vi "send load from string.vi"(8 "error in":errorcluster, 9 "target index":i32, 10 "system data":string, 11 "message queue in":T1) -> (0 "error out":errorcluster, 3 "message queue out":T1)   [LabVIEW 2013, in "module execution process.lvlib"]
uses:
  module execution process.lvlib
  <vilib>/NI/AMC/Message Queue.ctl
  <vilib>/NI/AMC/Message.ctl
  <vilib>/NI/Tools/Keyed Array/KeyedArray.ctl
  command commands to rtexe process.ctl
  <vilib>/NI/AMC/Create Single Message.vi
  <vilib>/NI/AMC/Update Message Routing Info.vi
  <vilib>/NI/AMC/Send Message.vi
  <vilib>/NI/AMC/AMC.lvlib
  <vilib>/NI/Tools/Keyed Array/Tools_KeyedArray.lvlib
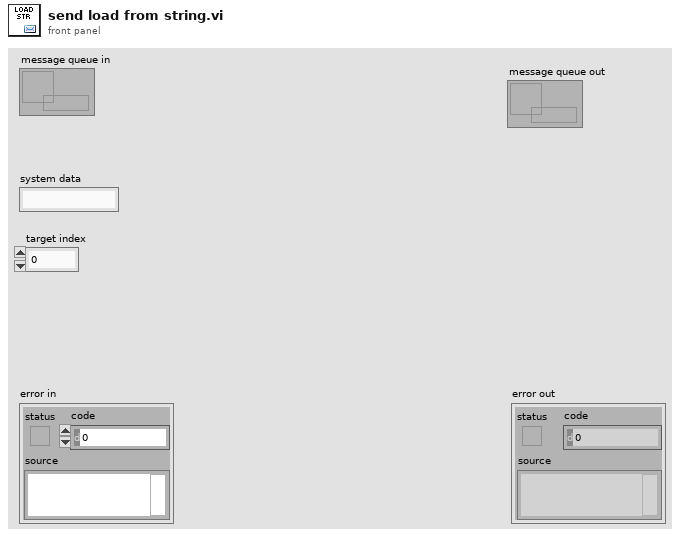
[diagram p1: front panel]
types:
  T1 = typedef "AMC.lvlib/Message Queue.ctl" = refnum<queue>
  T2 = typedef "module execution process.lvlib/command commands to rtexe process.ctl" = enum16{"Initialize", "Load from File", "Load from String", "Open All Engines", "Open Single Engine", "Initialize All Engines", "Initialize Single Engine", "Start All", "Start Single", "Pause All", "Pause Single", "Stop All", "Stop Single", "Close All", "Close Single", "Set Safe State All", "Set Safe State Single", "Get Status", "Exit", "Error", "Load Bitfile", "Unload Bitfile", "Add Search Paths"}
  T3 = cluster{"system data":string, "target index":i32}
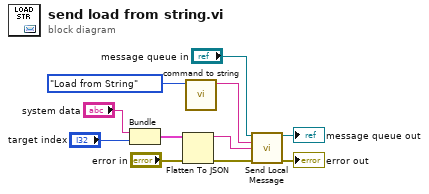
[diagram p0: block diagram]
diagram:
  n1 = Bundle("system data"="system data", "target index"="target index") -> (w2:T3)  [unwired: 1 in]
  n2 = Flatten To JSON(anything=w2, error in (no error)="error in") -> (JSON string=w4:string, 11:w5:errorcluster)  [unwired: 1 in]
  n3 = call "command to string.vi"("commands"=command_commands_to_rtexe_process."Load from String") -> ("command string"=w7:string)  [unwired: 10 in]
  n4 = call <vilib>:"Send Local Message.vi"("message queue in"="message queue in", "message name"=w7, "message value"=w4, "error in"=w5) -> ("message queue out"=→"message queue out":T1, "error out"=→"error out":errorcluster)  [unwired: 9 in, 1 out]
